vi "sendTCPRequest.vi"(9 "Force Reset":bool, 10 "Data code":string, 11 "TCP Network Connection in":refnum<k5>) -> (2 "Connection Out":refnum<k5>, 3 "error out":errorcluster)   [LabVIEW 2016]
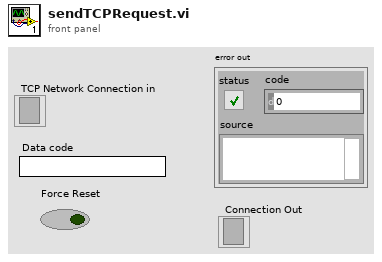
[diagram p1: front panel]
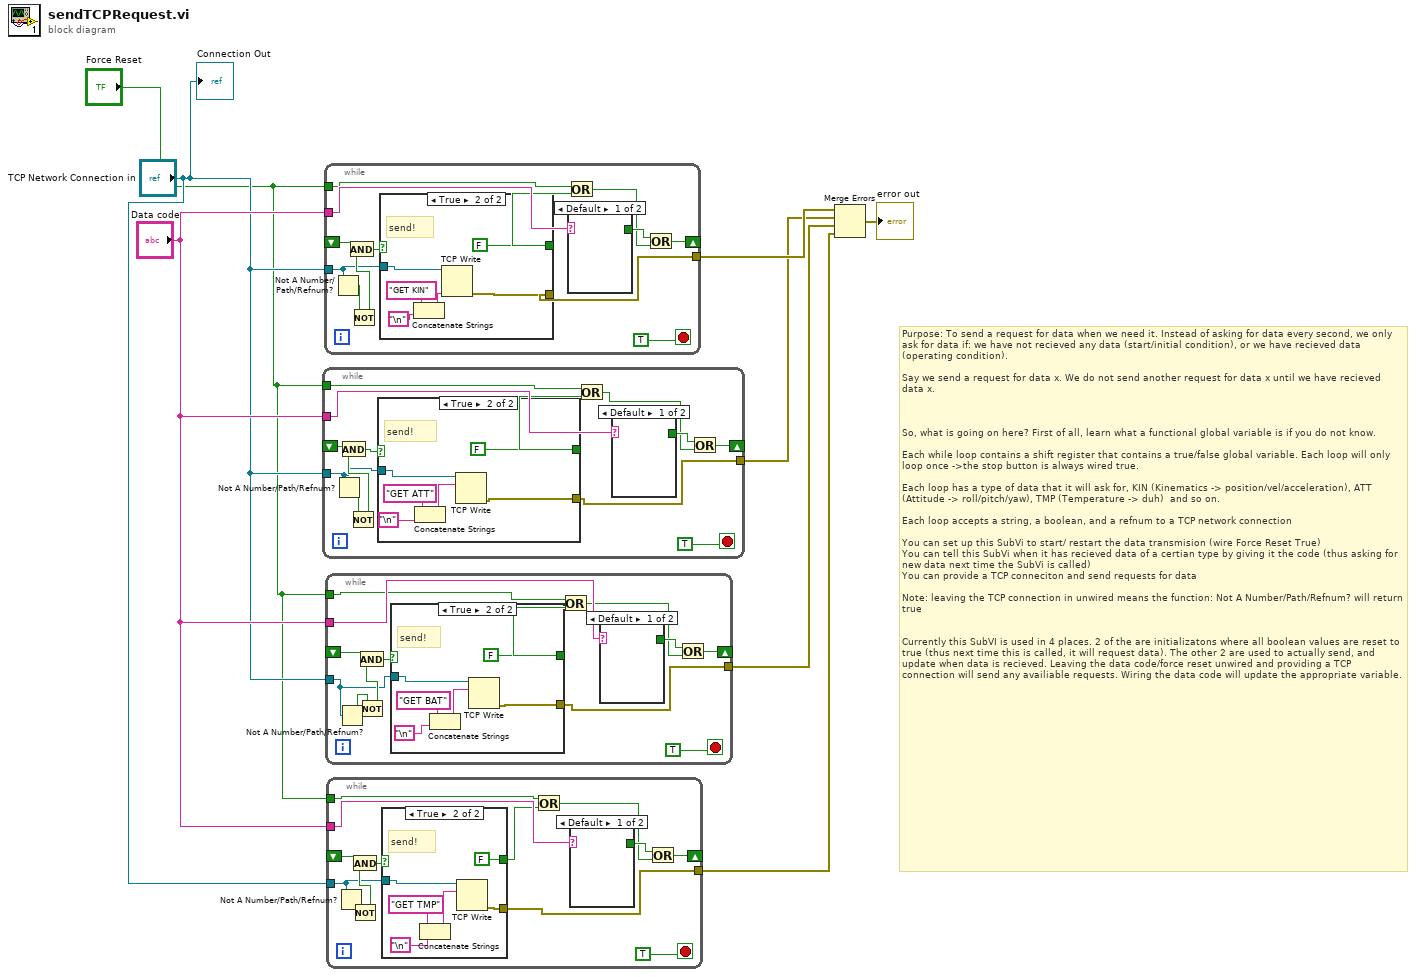
[diagram p0: block diagram]
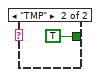
[diagram p3: hidden frame]
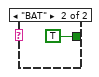
[diagram p5: hidden frame]
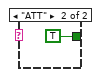
[diagram p7: hidden frame]
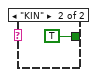
[diagram p9: hidden frame]
diagram:
  # "Purpose: To send a request for data when we need it. Instead of asking for data every second, we only ask for data if: we have not recieved any data (start/initial condition), or we have recieved data (operating condition). \n\nSay we send a request for data x. We do not send another request for data x until we have recieved data x.\n\n\n\nSo, what is going on here? First of all, learn what a functional global variable is if you do not know. \n\nEach while loop contains a shift register that contains a true/false global variable. Each loop will only loop once ->the stop button is always wired true. \n\nEach loop has a type of data that it will ask for, KIN (Kinematics -> position/vel/acceleration), ATT (Attitude -> roll/pitch/yaw), TMP (Temperature -> duh)  and so on. \n\nEach loop accepts a string, a boolean, and a refnum to a TCP network connection\n\nYou can set up this SubVi to start/ restart the data transmision (wire Force Reset True)\nYou can tell this SubVi when it has recieved data of a certian type by giving it the code (thus asking for new data next time the SubVi is called)\nYou can provide a TCP conneciton and send requests for data\n\nNote: leaving the TCP connection in unwired means the function: Not A Number/Path/Refnum? will return true\n\n\nCurrently this SubVI is used in 4 places. 2 of the are initializatons where all boolean values are reset to true (thus next time this is called, it will request data). The other 2 are used to actually send, and update when data is recieved. Leaving the data code/force reset unwired and providing a TCP connection will send any availiable requests. Wiring the data code will update the appropriate variable."
  n1 = while {
    shift-right: [w17] -> _
    shift-left: _ -> [w11]
    tunnel: "Data code" -> [w21]
    tunnel: "TCP Network Connection in" -> [w9]
    tunnel: [w19] -> w5
    tunnel: "Force Reset" -> [w14]
    stop <- TRUE stop-if-true
    n2 = Not A Number/Path/Refnum?(number/path/refnum=w9) -> (NaN/Path/Refnum?=w13:bool)
    n3 = Not(x=w13) -> (.not. x?=w12:bool)
    n4 = And(x=w11, y=w12) -> (x .and. y?=w10:bool)
    n5 = case shown="True" w10 {
      selector: w10 -> [w22 _]
      tunnel: w9 -> [_ w28]
      tunnel: [_ w27] -> w19
      tunnel: [w22 FALSE] -> w16
      frame False {
      }
      frame True {
        # "send!"
        n6 = Concatenate Strings("GET ATT", "\n") -> (w23:string)
        n7 = TCP Write(connection ID=w28, data in=w23) -> (error out=w27:errorcluster)  [unwired: 2 in, 2 out]
      }
    }
    n8 = Or(x=w14, y=w16) -> (x .or. y?=w15:bool)
    n9 = case shown="Default" w21 {
      tunnel: [_ TRUE] -> w18
      frame Default {
      }
      frame "ATT" {
      }
    }
    n10 = Or(x=w18, y=w15) -> (x .or. y?=w17:bool)
  }
  n11 = while {
    shift-right: [w38] -> _
    shift-left: _ -> [w32]
    tunnel: "Data code" -> [w42]
    tunnel: "TCP Network Connection in" -> [w30]
    tunnel: [w40] -> w8
    tunnel: "Force Reset" -> [w35]
    stop <- TRUE stop-if-true
    n12 = Not A Number/Path/Refnum?(number/path/refnum=w30) -> (NaN/Path/Refnum?=w34:bool)
    n13 = Not(x=w34) -> (.not. x?=w33:bool)
    n14 = And(x=w32, y=w33) -> (x .and. y?=w31:bool)
    n15 = case shown="True" w31 {
      selector: w31 -> [w43 _]
      tunnel: w30 -> [_ w49]
      tunnel: [_ w48] -> w40
      tunnel: [w43 FALSE] -> w37
      frame False {
      }
      frame True {
        # "send!"
        n16 = Concatenate Strings("GET KIN", "\n") -> (w44:string)
        n17 = TCP Write(connection ID=w49, data in=w44) -> (error out=w48:errorcluster)  [unwired: 2 in, 2 out]
      }
    }
    n18 = Or(x=w35, y=w37) -> (x .or. y?=w36:bool)
    n19 = case shown="Default" w42 {
      tunnel: [_ TRUE] -> w39
      frame Default {
      }
      frame "KIN" {
      }
    }
    n20 = Or(x=w39, y=w36) -> (x .or. y?=w38:bool)
  }
  n21 = while {
    shift-right: [w59] -> _
    shift-left: _ -> [w54]
    tunnel: "Data code" -> [w63]
    tunnel: "TCP Network Connection in" -> [w52]
    tunnel: [w61] -> w4
    tunnel: "Force Reset" -> [w56]
    stop <- TRUE stop-if-true
    n22 = Not A Number/Path/Refnum?(number/path/refnum=w52) -> (NaN/Path/Refnum?=w53:bool)
    n23 = Not(x=w53) -> (.not. x?=w55:bool)
    n24 = And(x=w54, y=w55) -> (x .and. y?=w51:bool)
    n25 = case shown="True" w51 {
      selector: w51 -> [w64 _]
      tunnel: w52 -> [_ w70]
      tunnel: [_ w69] -> w61
      tunnel: [w64 FALSE] -> w58
      frame False {
      }
      frame True {
        # "send!"
        n26 = Concatenate Strings("GET BAT", "\n") -> (w65:string)
        n27 = TCP Write(connection ID=w70, data in=w65) -> (error out=w69:errorcluster)  [unwired: 2 in, 2 out]
      }
    }
    n28 = Or(x=w56, y=w58) -> (x .or. y?=w57:bool)
    n29 = case shown="Default" w63 {
      tunnel: [_ TRUE] -> w60
      frame Default {
      }
      frame "BAT" {
      }
    }
    n30 = Or(x=w60, y=w57) -> (x .or. y?=w59:bool)
  }
  n31 = while {
    shift-right: [w80] -> _
    shift-left: _ -> [w75]
    tunnel: "Data code" -> [w84]
    tunnel: "TCP Network Connection in" -> [w72]
    tunnel: [w82] -> w3
    tunnel: "Force Reset" -> [w77]
    stop <- TRUE stop-if-true
    n32 = Not A Number/Path/Refnum?(number/path/refnum=w72) -> (NaN/Path/Refnum?=w73:bool)
    n33 = Not(x=w73) -> (.not. x?=w76:bool)
    n34 = And(x=w75, y=w76) -> (x .and. y?=w74:bool)
    n35 = case shown="True" w74 {
      selector: w74 -> [w85 _]
      tunnel: w72 -> [_ w91]
      tunnel: [_ w90] -> w82
      tunnel: [w85 FALSE] -> w79
      frame False {
      }
      frame True {
        # "send!"
        n36 = Concatenate Strings("GET TMP", "\n") -> (w86:string)
        n37 = TCP Write(connection ID=w91, data in=w86) -> (error out=w90:errorcluster)  [unwired: 2 in, 2 out]
      }
    }
    n38 = Or(x=w77, y=w79) -> (x .or. y?=w78:bool)
    n39 = case shown="Default" w84 {
      tunnel: [_ TRUE] -> w81
      frame Default {
      }
      frame "TMP" {
      }
    }
    n40 = Or(x=w81, y=w78) -> (x .or. y?=w80:bool)
  }
  n41 = Merge Errors(w8, w5, w4, w3) -> (→"error out":errorcluster)
  "Connection Out" <- "TCP Network Connection in"
